vi "Build Report String.vi"(8 "error in (no error)":errorcluster, 10 "Result":T1, 11 "Action Step in":refnum<class "Action Step.lvclass">) -> (0 "error out":errorcluster, 2 "Report String":string, 3 "Action Step out":refnum<class "Action Step.lvclass">)   [LabVIEW 2020, in "MacroAssert.lvlib" / "Action Step.lvclass"]
doc: "Builds a string using <B>Step</B> and <B>Result</B> to be included in a report."
uses:
  Action Step.lvclass
  Action Step.lvclass/Action Step.ctl
  MacroAssert.lvlib
  CTLs/Result.ctl
  CTLs/Outcome.ctl
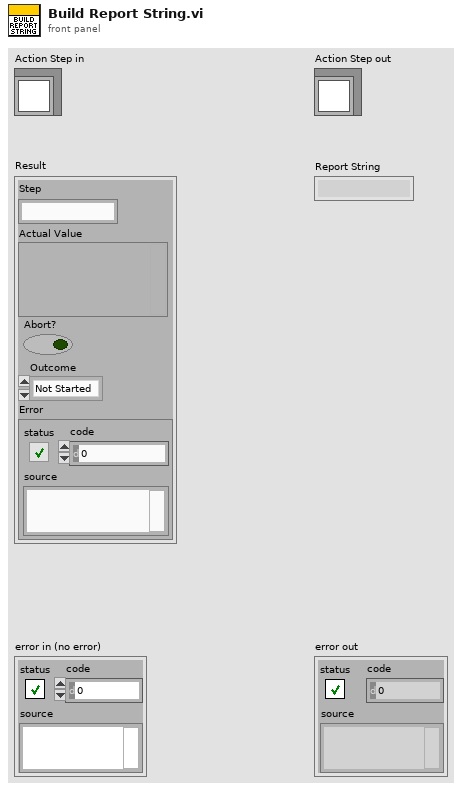
[diagram p1: front panel]
types:
  T1 = typedef "MacroAssert.lvlib/Result.ctl" = cluster{"Step":string, "Actual Value":variant, "Abort?":bool, "Outcome":T2, "Error":errorcluster}
  T2 = typedef "MacroAssert.lvlib/Outcome.ctl" = enum16{"Not Started", "Skipped", "Pass", "Fail", "Complete", "Error", "Auto Abort", "User Abort"}
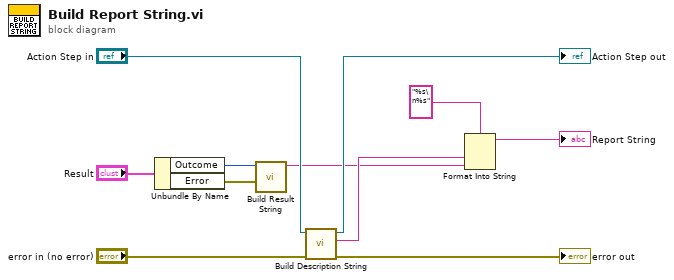
[diagram p0: block diagram]
diagram:
  n1 = Unbundle By Name("Result") -> ("Outcome"=w3:T2, "Error"=w2:errorcluster)
  n2 = call "Build Result String.vi"("Error"=w2, "Outcome"=w3) -> ("Result String"=w1:string)  [unwired: 9 in]
  n3 = call-dynamic "Build Description String.vi"("error in (no error)"="error in (no error)", "Action Step in"="Action Step in") -> ("error out"=→"error out":errorcluster, "Description"=w6:string, "Action Step out"=→"Action Step out":refnum<class "Action Step.lvclass">)  [unwired: 7 in]
  n4 = Format Into String(format string="%s\n%s", w6, w1) -> (resulting string=→"Report String":string)  [unwired: 2 in, 1 out]
